vi "G#Object_ErrorMissingMethod.vi"(0 "reference in":refnum<class "G#Object.lvclass">, 5 "error in (no error)":errorcluster, 7 "call depth (1)":i32=1) -> (14 "reference out":refnum<class "G#Object.lvclass">, 19 "error out":errorcluster)   [LabVIEW 2020, in "G#Object.lvclass"]
doc: "Sets an error to indicate that a abstract method is not implemented."
uses:
  G#Object.lvclass
  G#Object.lvclass/G#Object.ctl
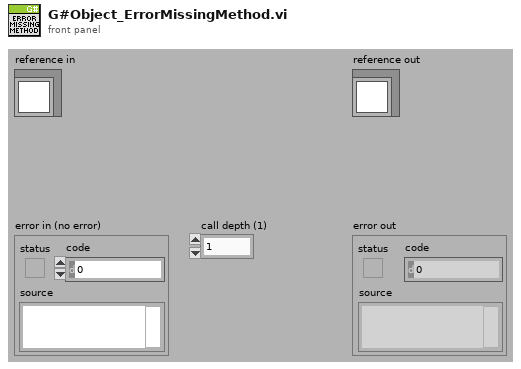
[diagram p1: front panel]
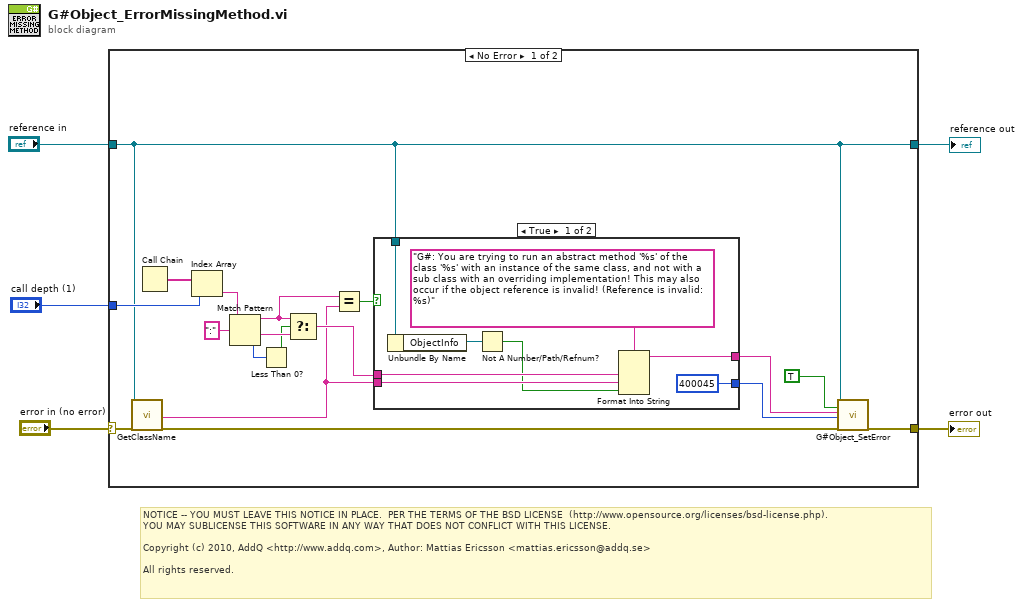
[diagram p0: block diagram]
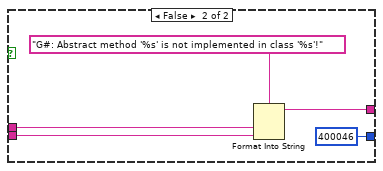
[diagram p2: hidden frame]
diagram:
  # "NOTICE -- YOU MUST LEAVE THIS NOTICE IN PLACE.  PER THE TERMS OF THE BSD LICENSE  (http://www.opensource.org/licenses/bsd-license.php).\nYOU MAY SUBLICENSE THIS SOFTWARE IN ANY WAY THAT DOES NOT CONFLICT WITH THIS LICENSE.\n\nCopyright (c) 2010, AddQ <http://www.addq.com>, Author: Mattias Ericsson <mattias.ericsson@addq.se>\n\nAll rights reserved."
  n1 = case shown="No Error" "error in (no error)" {
    selector: "error in (no error)" -> [w14 w38]
    tunnel: [w16 w38] -> w1
    tunnel: "call depth (1)" -> [w15 _]
    tunnel: "reference in" -> [w6 w37]
    tunnel: [w6 w37] -> w3
    frame No Error {
      n2 = call-dynamic "GetClassName.vi"("reference in"=w6, "error in (no error)"=w14) -> ("full class name"=w7:string, "error out"=w13:errorcluster)  [unwired: 13 in, 3 out]
      n3 = Call Chain() -> (call chain=w18:string[])
      n4 = Index Array(array=w18, index=w15) -> (element=w17:string)
      n5 = Match Pattern(string=w17, regular expression=":") -> (before substring=w8:string, after substring=w22:string, offset past match=w21:i32)  [unwired: 2 out]
      n6 = Less Than 0?(x=w21) -> (x < 0?=w20:bool)
      n7 = Select(t=w8, s=w20, f=w22) -> (s? t:f=w11:string)
      n8 = Equal?(x=w8, y=w7) -> (x = y?=w10:bool)
      n9 = case shown="True" w10 {
        tunnel: [w31 w35] -> w19
        tunnel: w11 -> [w30 w34]
        tunnel: w7 -> [w29 w33]
        tunnel: [400045 ("ErrorCode(5000)") 400046 ("ErrorCode(5000)")] -> w9
        tunnel: w6 -> [w27 _]
        frame True {
          n10 = Unbundle By Name(w27) -> ("ObjectInfo"=w26:refnum<queue>)
          n11 = Not A Number/Path/Refnum?(number/path/refnum=w26) -> (NaN/Path/Refnum?=w24:bool)
          n12 = Format Into String(format string="G#: You are trying to run an abstract method '%s' of the class '%s' with an instance of the same class, and not with a sub class with an overriding implementation! This may also occur if the object reference is invalid! (Reference is invalid: %s)", w30, w29, w24) -> (resulting string=w31:string)  [unwired: 2 in, 1 out]
        }
        frame False {
          n13 = Format Into String(format string="G#: Abstract method '%s' is not implemented in class '%s'!", w34, w33) -> (resulting string=w35:string)  [unwired: 2 in, 1 out]
        }
      }
      n14 = call "G#Object_SetError.vi"("reference in"=w6, "error (F)"=TRUE ("error"), "source"=w19, "code"=w9, "error in (no error)"=w13) -> ("error out"=w16:errorcluster)  [unwired: 14 in]
    }
    frame Error {
    }
  }
  "reference out" <- w3
  "error out" <- w1
